vi "NF WF1973_74 TRAC XY.vi"(0 "VISAsession":refnum<visa-resource-name>, 1 "Point(4096)":i32=4096 min=0 max=10000 step=1, 2 "Function(Sin)":u16(ring) items=["Sin", "Sin(x)/x", "Clear"], 5 "Memory No.(0)":u16 max=128 step=1, 7 "Name(USER)":string="USER", 9 "Level":dbl(knob)=1.0 min=0.0 max=1.0 step=0.01 scale=0.0..1.0 scale format="%.2f", 11 "Error IN":errorcluster, 12 "Read(F)":bool) -> (4 "CopyVISAsession":refnum<visa-resource-name>, 15 "Error OUT":errorcluster)   [LabVIEW 2010]
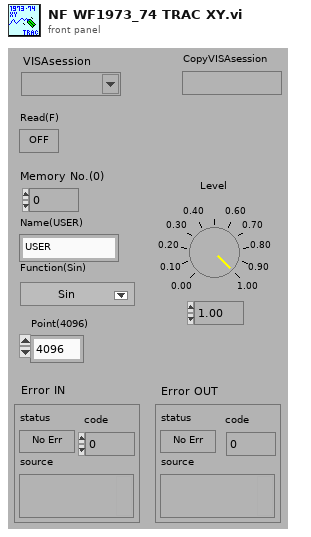
[diagram p1: front panel]
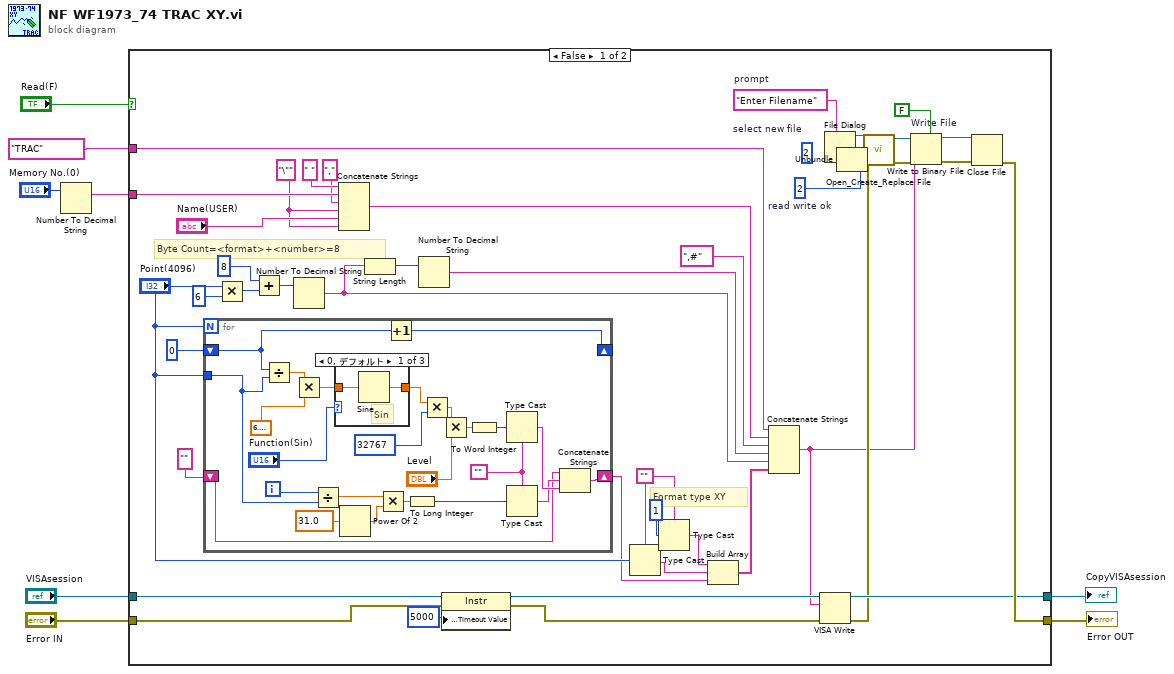
[diagram p0: block diagram]
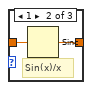
[diagram p2: hidden frame]
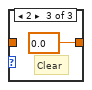
[diagram p3: hidden frame]
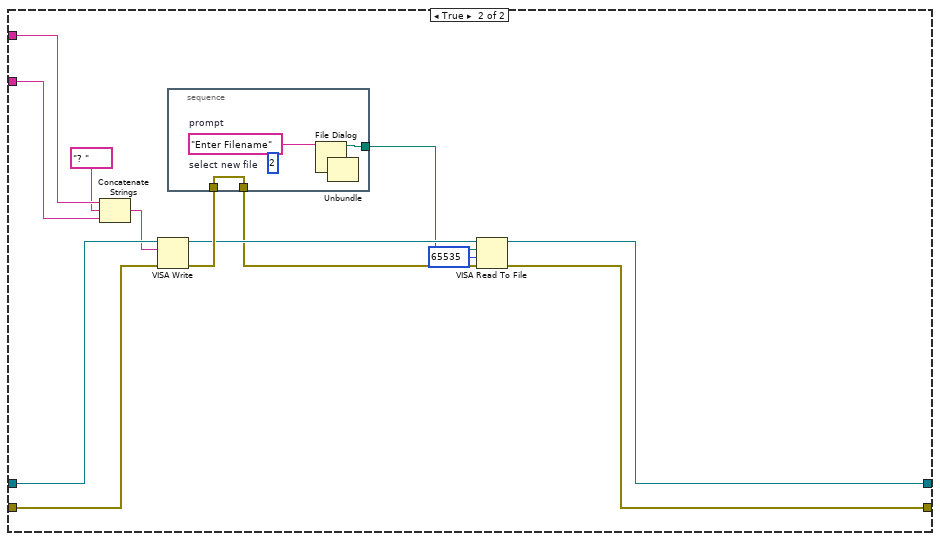
[diagram p4: hidden frame]
diagram:
  n1 = Number To Decimal String(number="Memory No.(0)") -> (decimal integer string=w1:string)  [unwired: 1 in]
  n2 = case shown="FALSE" "Read(F)" {
    tunnel: [w42 w80] -> w8
    tunnel: [w43 w85] -> w7
    tunnel: "VISAsession" -> [w22 w92]
    tunnel: "Error IN" -> [w20 w91]
    tunnel: "TRAC" -> [w40 w89]
    tunnel: w1 -> [w31 w87]
    frame False {
      w25 = "\""
      w16 = ""
      w50 = "Enter Filename"  # prompt
      w44 = 2  # read write ok
      (unwired) i16 2  # select new file
      # "Format type XY"
      # "Byte Count=<format>+<number>=8"
      n3 = for {
        N: "Point(4096)" -> [_]
        shift-right: [w71] -> _
        shift-left: u16 0 -> [w72]
        tunnel: "Point(4096)" -> [w56]
        shift-right: [w59] -> w13
        shift-left: "" -> [w58]
        i -> [w55]
        w60 = ""
        n4 = Divide(x=w72, y=w56) -> (x/y=w74:dbl)
        n5 = Multiply(x=w74, y=6.283185307179586) -> (x*y=w70:dbl)
        n6 = Divide(x=w55, y=w56) -> (x/y=w68:dbl)
        n7 = case shown="0, デフォルト" "Function(Sin)" {
          tunnel: w70 -> [w76 w78 _]
          tunnel: [w75 w77 0.0] -> w57
          frame 0, Default {
            # "Sin"
            n8 = Sine(x=w76) -> (sin(x)=w75:dbl)
          }
          frame 1 {
            # "Sin(x)/x"
            n9 = Sinc(1:w78) -> (0:w77:dbl)
          }
          frame 2 {
            # "Clear"
          }
        }
        n10 = Power Of 2(x=31.0) -> (2^x=w67:dbl)
        n11 = Multiply(x=w68, y=w67) -> (x*y=w65:dbl)
        n12 = Increment(x=w72) -> (x+1=w71:u16)
        n13 = To Long Integer(number=w65) -> (32bit integer=w63:i32)
        n14 = Multiply(x=w57, y=32767) -> (x*y=w53:dbl)
        n15 = Multiply(x=w53, y="Level") -> (x*y=w54:dbl)
        n16 = To Word Integer(number=w54) -> (16bit integer=w64:i16)
        n17 = Type Cast(type=w60, x=w64) -> (*(type *) &x=w62:string)
        n18 = Type Cast(type=w60, x=w63) -> (*(type *) &x=w61:string)
        n19 = Concatenate Strings(w58, w61, w62) -> (w59:string)
      }
      n20 = Multiply(x="Point(4096)", y=6) -> (x*y=w38:i32)
      n21 = Add(x=8, y=w38) -> (x+y=w36:i32)
      n22 = Number To Decimal String(number=w36) -> (decimal integer string=w32:string)  [unwired: 1 in]
      n23 = Concatenate Strings(" ", w31, ",", w25, "Name(USER)", w25) -> (w28:string)
      n24 = String Length(string=w32) -> (length=w35:i32)
      n25 = Number To Decimal String(number=w35) -> (decimal integer string=w33:string)  [unwired: 1 in]
      n26 = property class="Instr"(reference=w22, error in=w20, "General Settings:Timeout Value"=u32 5000) -> (reference out=w23:refnum<visa-resource-name>, error out=w21:errorcluster)
      n27 = Type Cast(type=w16, x="Point(4096)") -> (*(type *) &x=w15:string)
      n28 = Type Cast(type=w16, x=1) -> (*(type *) &x=w17:string)
      n29 = Build Array(w17, w15, w13) -> (w19:string[])
      n30 = Concatenate Strings(w40, w28, ",#", w33, w32, w19) -> (w11:string)
      n31 = VISA Write(VISA resource name=w23, write buffer=w11, error in (no error)=w21) -> (VISA resource name out=w42:refnum<visa-resource-name>, error out=w41:errorcluster)  [unwired: 1 out]
      n32 = File Dialog(7:w50) -> (0:w10:errorcluster, 3:w47:path)  [unwired: 6 in, 2 out]
      n33 = Unbundle(w10) -> ()  [unwired: 3 out]
      n34 = call <vilib>:"Open_Create_Replace File.vi"("error in (no error)"=w41, "function (open:0)"=w44, "file path"=w47) -> ("error out"=w45:errorcluster, "refnum"=w46:refnum<file>)  [unwired: 5 in, 2 out]
      n35 = Write to Binary File "Write File"(file (use dialog)=w46, data=w11, error in=w45, 5:FALSE ("配列または文字列サイズを先頭に追加?（T）")) -> (refnum out=w49:refnum<file>, error out=w48:errorcluster)  [unwired: 2 in, 1 out]
      n36 = Close File(refnum=w49, error in=w48) -> (error out=w43:errorcluster)  [unwired: 1 out]
    }
    frame True {
      n37 = Concatenate Strings(w89, "? ", w87) -> (w90:string)
      n38 = VISA Write(VISA resource name=w92, write buffer=w90, error in (no error)=w91) -> (VISA resource name out=w84:refnum<visa-resource-name>, error out=w86:errorcluster)  [unwired: 1 out]
      n39 = stacked-sequence {
        tunnel: [w95] -> w81
        tunnel: w86 -> [w94]
        tunnel: [w94] -> w83
        frame #0 {
          w96 = "Enter Filename"  # prompt
          (unwired) i16 2  # select new file
          n40 = File Dialog(7:w96) -> (0:w93:errorcluster, 3:w95:path)  [unwired: 6 in, 2 out]
          n41 = Unbundle(w93) -> ()  [unwired: 3 out]
        }
      }
      n42 = VISA Read To File(8:w83, 9:u32 65535 ("カウント (1024)"), 10:w81, 11:w84) -> (0:w85:errorcluster, 3:w80:refnum<visa-resource-name>)  [unwired: 1 out]
    }
  }
  "CopyVISAsession" <- w8
  "Error OUT" <- w7
